vi "Start Download.vi"(8 "Error In":errorcluster, 10 "Download Directory":path, 11 "URL":string) -> (0 "Error Out":errorcluster, 3 "Download":T1)   [LabVIEW 2014, in "LMH-Toolbox.lvlib"]
doc: "Start downloading the file specified by the URL input."
uses:
  <vilib>/MakerHub/Toolbox/LMH-Toolbox.lvlib
  <vilib>/MakerHub/Toolbox/Private/Web/Type Defs/Download Task.ctl
  <vilib>/regexp/Match Regular Expression.xnode
  <vilib>/MakerHub/Toolbox/Private/Web/LMH-Web.lvlib
  <vilib>/httpClient/LabVIEWHTTPClient.lvlib
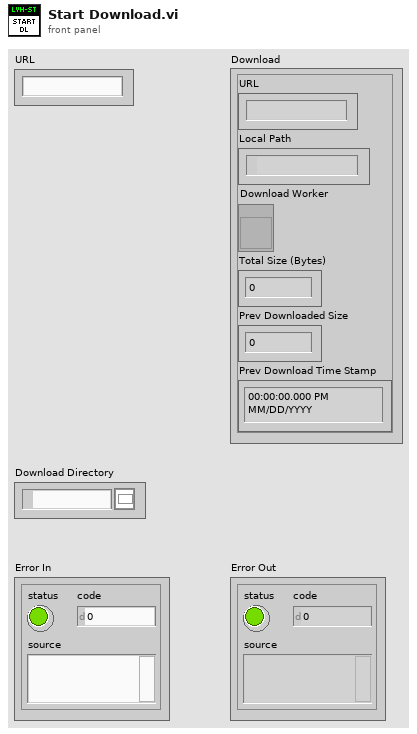
[diagram p1: front panel]
types:
  T1 = typedef "LMH-Toolbox.lvlib/LMH-Web.lvlib/Download Task.ctl" = cluster{"URL":string, "Local Path":path, "Download Worker":refnum<vi>, "Total Size (Bytes)":u64, "Prev Downloaded Size":u64, "Prev Download Time Stamp":timestamp}
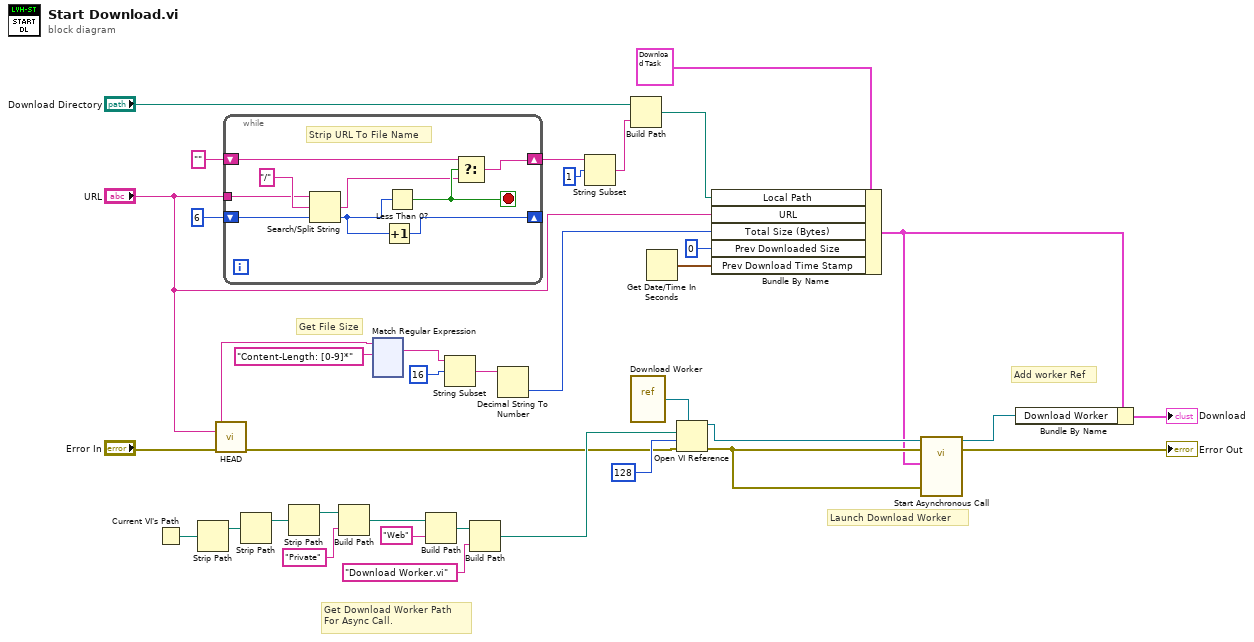
[diagram p0: block diagram]
diagram:
  # "Add worker Ref"
  # "Launch Download Worker"
  # "Get File Size"
  # "Get Download Worker Path \nFor Async Call."
  n1 = Current VI's Path() -> (path=w1:path)
  n2 = Strip Path(path=w1) -> (stripped path=w2:path)  [unwired: 1 out]
  n3 = call <vilib>:"HEAD.vi"("url"="URL", "error in (no error)"="Error In") -> ("headers"=w11:string, "error out"=w16:errorcluster)  [unwired: 11 in, 1 out]
  n4 = while {
    shift-right: [w43] -> _
    shift-left: 6 ("offset (0)") -> [w45]
    shift-right: [w40] -> w31
    shift-left: "" ("search string/char (-)") -> [w41]
    tunnel: "URL" -> [w38]
    stop <- w42 stop-if-true
    # "Strip URL To File Name"
    n5 = Search/Split String(string=w38, search string/char (-)="/", offset (0)=w45) -> (match + rest of string=w39:string, offset of match=w44:i32)  [unwired: 1 out]
    n6 = Increment(x=w44) -> (x+1=w43:i32)
    n7 = Less Than 0?(x=w44) -> (x < 0?=w42:bool)
    n8 = Select(t=w41, s=w42, f=w39) -> (s? t:f=w40:string)
  }
  n9 = Strip Path(path=w2) -> (stripped path=w26:path)  [unwired: 1 out]
  n10 = Strip Path(path=w26) -> (stripped path=w25:path)  [unwired: 1 out]
  n11 = Build Path(base path=w25, name or relative path="Private") -> (appended path=w24:path)
  n12 = xnode "Match Regular Expression"("input string"=w11, "regular expression"="Content-Length: [0-9]*") -> ("whole match"=w15:string)  [unwired: 4 in, 4 out]
  n13 = Build Path(base path=w24, name or relative path="Web") -> (appended path=w21:path)
  n14 = String Subset(string=w15, offset (0)=16) -> (substring=w13:string)  [unwired: 1 in]
  n15 = Build Path(base path=w21, name or relative path="Download Worker.vi") -> (appended path=w19:path)
  n16 = Decimal String To Number(string=w13) -> (number=w10:i32)  [unwired: 2 in, 1 out]
  n17 = String Subset(string=w31, offset (0)=1) -> (substring=w27:string)  [unwired: 1 in]
  n18 = Build Path(base path="Download Directory", name or relative path=w27) -> (appended path=w6:path)
  n19 = vi-ref <vilib>:"Download Worker.vi"() -> (w36:refnum<vi>)
  n20 = Get Date/Time In Seconds() -> (seconds since 1Jan1904=w8:timestamp)
  n21 = Open VI Reference(type specifier VI Refnum (for type only)=w36, vi path=w19, options=128, error in (no error)=w16) -> (vi reference=w33:refnum<vi>, error out=w34:errorcluster)  [unwired: 2 in]
  n22 = Bundle By Name(cluster=T1 {"URL"="", "Local Path"=path "", "Download Worker"=refnum, "Total Size (Bytes)"=0, "Prev Downloaded Size"=0, "Prev Download Time Stamp"=timestamp(0 s since 1904-01-01)} ("Download"), "Local Path"=w6, "URL"="URL", "Total Size (Bytes)"=w10, "Prev Downloaded Size"=u64 0, "Prev Download Time Stamp"=w8) -> (w5:T1)
  n23 = call-by-ref "Start Asynchronous Call"(reference=w33, error in=w34, "Error In"=w34, "Download"=w5) -> (reference out=w4:refnum<vi>, error out=→"Error Out":errorcluster)  [unwired: 8 in, 2 out]
  n24 = Bundle By Name(cluster=w5, "Download Worker"=w4) -> (→"Download":T1)
